vi "chart series set invert if negative.vi"(8 "error in (no error)":errorcluster, 11 "series":u32) -> (0 "error out":errorcluster)   [LabVIEW 2015, in "xlsxwriter.lvlib"]
doc: "void chart_series_set_invert_if_negative(lxw_chart_series series);"
uses:
  xlsxwriter.lvlib
  xlsxwriter.dll
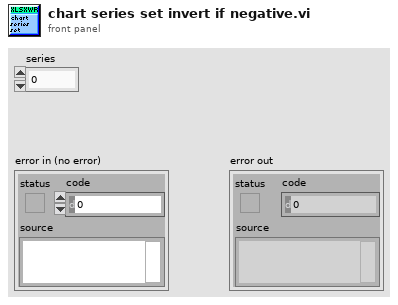
[diagram p1: front panel]
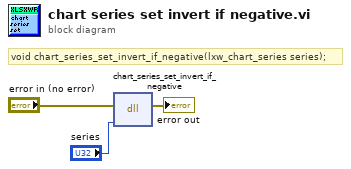
[diagram p0: block diagram]
diagram:
  # "void chart_series_set_invert_if_negative(lxw_chart_series series);"
  n1 = dll-call lib="C:/Users/WDAGUtilityAccount/Desktop/lv_vis_added_cell/xlsxwriter.*" fn="chart_series_set_invert_if_negative"(error in="error in (no error)", "series"="series") -> (error out=→"error out":errorcluster)  [unwired: 4 in, 1 out]
